vi "Add Comment.vi"(8 "Error In":errorcluster) -> (0 "Error Out":errorcluster, 2 "Comment out":string, 3 "Commentor out":string, 5 "Add?":bool)   [LabVIEW 2014]
doc: "This VI allows user to import comment."
panel:
  in  "Enum":enum16{"idle", "add", "cancel"}(ring)
  in  "Cancel":bool
  in  "Add":bool
  in  "Commentor":string
  in  "Comment":string
  # "Add comment to the last configuration"
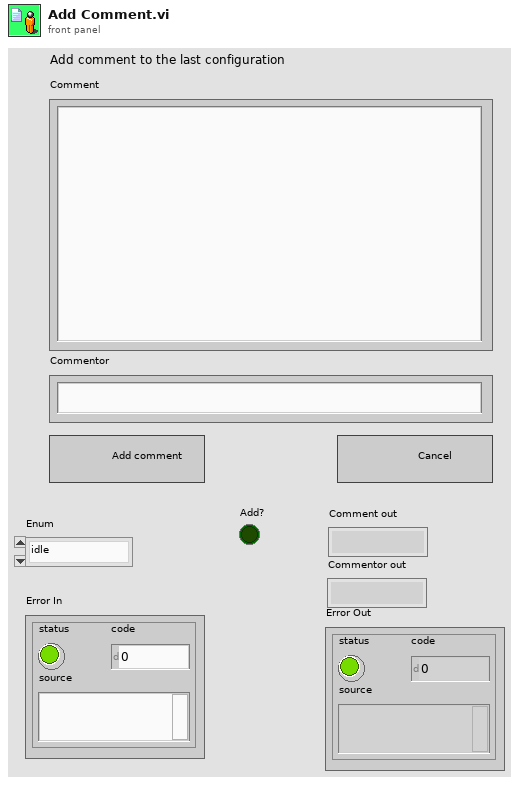
[diagram p1: front panel]
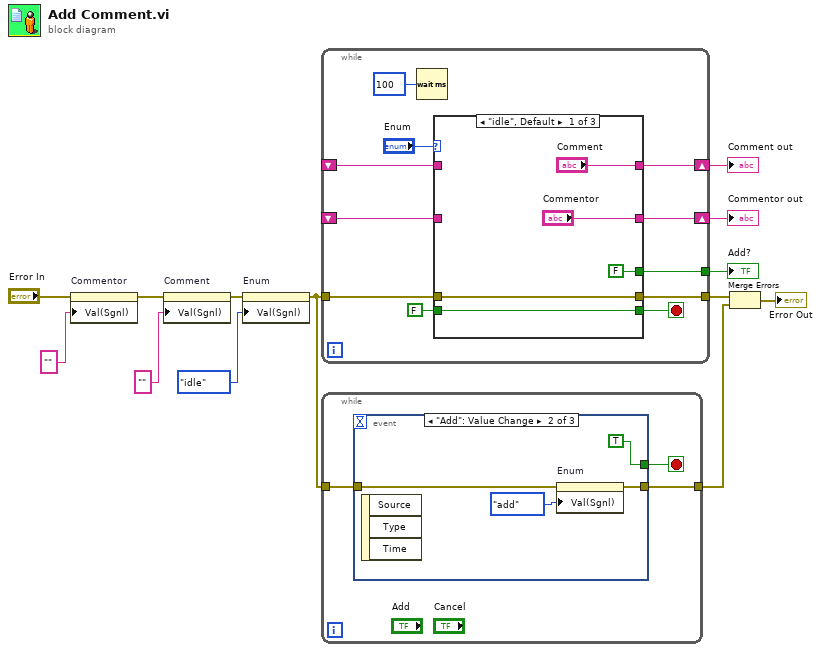
[diagram p0: block diagram]
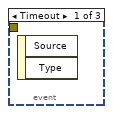
[diagram p2: hidden frame]
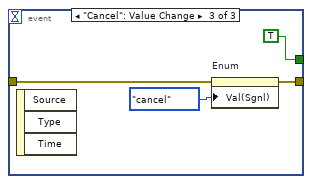
[diagram p3: hidden frame]
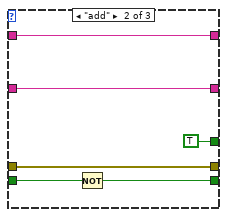
[diagram p4: hidden frame]
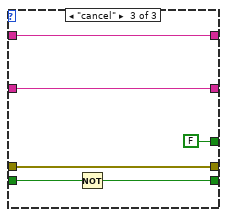
[diagram p5: hidden frame]
diagram:
  n1 = property on="Commentor" class="Str"(error in="Error In", "Val(Sgnl)"="" ("Value (Signaling)")) -> (error out=w3:errorcluster)  [unwired: 1 in, 1 out]
  n2 = property on="Comment" class="Str"(error in=w3, "Val(Sgnl)"="" ("Value (Signaling)")) -> (error out=w5:errorcluster)  [unwired: 1 in, 1 out]
  n3 = property on="Enum" class="Enum (strict)"(error in=w5, "Val(Sgnl)"=enum16{"idle", "add", "cancel"}."idle" ("Value (Signaling)")) -> (error out=w12:errorcluster)  [unwired: 1 in, 1 out]
  n4 = while {
    tunnel: w12 -> [w14]
    shift-right: [w22] -> w10
    shift-left: _ -> [w20]
    shift-right: [w21] -> w9
    shift-left: _ -> [w19]
    tunnel: [w16] -> w11
    tunnel: [w15] -> w8
    stop <- w17 stop-if-true
    n5 = Wait (ms)(milliseconds to wait=u32 100) -> ()  [unwired: 1 out]
    n6 = case shown="\"idle\", Default" "Enum" {
      tunnel: ["Comment" w35 w38] -> w22
      tunnel: ["Commentor" w34 w39] -> w21
      tunnel: w20 -> [_ w35 w38]
      tunnel: w19 -> [_ w34 w39]
      tunnel: FALSE -> [w27 w33 w41]
      tunnel: [w27 w32 w40] -> w17
      tunnel: [FALSE TRUE FALSE] -> w16
      tunnel: [w25 w30 w36] -> w15
      tunnel: w14 -> [w25 w30 w36]
      frame "idle", Default {
      }
      frame "add" {
        n7 = Not(x=w33) -> (.not. x?=w32:bool)
      }
      frame "cancel" {
        n8 = Not(x=w41) -> (.not. x?=w40:bool)
      }
    }
  }
  "Add?" <- w11
  "Comment out" <- w10
  "Commentor out" <- w9
  n9 = while {
    tunnel: w12 -> [w44]
    tunnel: [w43] -> w7
    stop <- w42 stop-if-true
    n10 = event shown="[1] \"Add\": Value Change" {
      selector: _ -> [_ _ _]
      dyn-events: _ -> [_ _ _]
      timeout: _ -> [_ _ _]
      tunnel: w44 -> [_ w48 w52]
      tunnel: [_ w46 w50] -> w43
      tunnel: [_ TRUE TRUE] -> w42
      event Timeout {
        n11 = event-data() -> ()  [unwired: 1 in, 2 out]
      }
      event "Add": Value Change {
        n12 = event-data() -> ()  [unwired: 1 in, 3 out]
        n13 = property on="Enum" class="Enum (strict)"(error in=w48, "Val(Sgnl)"=enum16{"idle", "add", "cancel"}."add" ("Value (Signaling)")) -> (error out=w46:errorcluster)  [unwired: 1 in, 1 out]
      }
      event "Cancel": Value Change {
        n14 = event-data() -> ()  [unwired: 1 in, 3 out]
        n15 = property on="Enum" class="Enum (strict)"(error in=w52, "Val(Sgnl)"=enum16{"idle", "add", "cancel"}."cancel" ("Value (Signaling)")) -> (error out=w50:errorcluster)  [unwired: 1 in, 1 out]
      }
    }
  }
  n16 = Merge Errors(w8, w7) -> (→"Error Out":errorcluster)
